vi "Configure Module.vi"(8 "error in (no error)":errorcluster, 10 "IOV ref in":refnum<k21>, 11 "Module Template in":refnum<class "9234.lvclass">) -> (0 "error out":errorcluster, 2 "IOV ref out":refnum<k21>, 3 "Module Template out":refnum<class "9234.lvclass">)   [LabVIEW 2017, in "Modules.lvlib" / "9234.lvclass"]
uses:
  9234.lvclass
  9234.lvclass/9234.ctl
  <resource>/objmgr/cRIO.rc
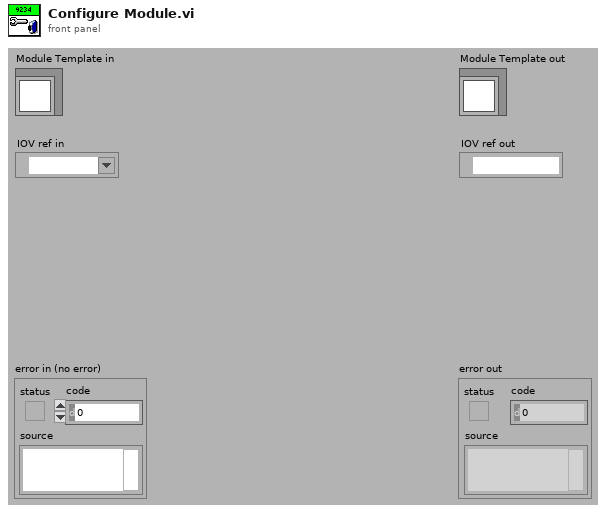
[diagram p1: front panel]
types:
  T1 = typedef "Modules.lvlib/9234.lvclass/Data rate.ctl" = u32
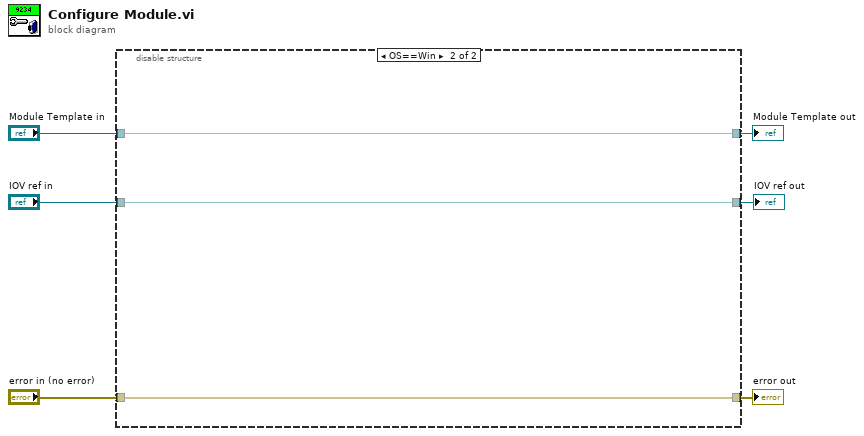
[diagram p0: block diagram]
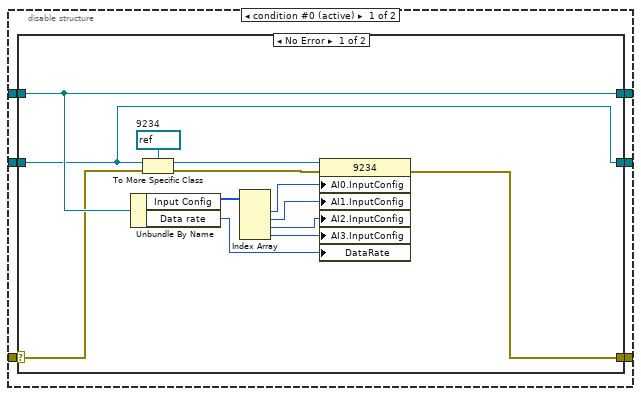
[diagram p2: hidden frame]
diagram:
  n1 = disable-structure shown="OS==Win" {
    disable-tunnel: "error in (no error)" -> [w12 w29]
    disable-tunnel: [w11 w29] -> w5
    disable-tunnel: "Module Template in" -> [w10 w31]
    disable-tunnel: [w9 w31] -> w3
    disable-tunnel: "IOV ref in" -> [w8 w30]
    disable-tunnel: [w7 w30] -> w1
    frame condition #0 (active) {
      n2 = case shown="No Error" w12 {
        selector: w12 -> [w24 w28]
        tunnel: [w20 w28] -> w11
        tunnel: [w25 w27] -> w9
        tunnel: w10 -> [w25 w27]
        tunnel: w8 -> [w19 w26]
        tunnel: [w19 w26] -> w7
        frame No Error {
          w23 = refnum<k21> refnum  # 9234
          n3 = Unbundle By Name(w25) -> ("Input Config"=w18:u32[], "Data rate"=w13:T1)
          n4 = To More Specific Class(target class=w23, reference=w19, error in=w24) -> (specific class reference=w22:refnum<k21>, error out=w21:errorcluster)
          n5 = Index Array(array=w18) -> (element #1=w17:u32, element #2=w16:u32, element #3=w15:u32, element #4=w14:u32)  [unwired: 4 in]
          n6 = property class="9234"(reference=w22, error in=w21, "AI0.InputConfig"=w17, "AI1.InputConfig"=w16, "AI2.InputConfig"=w15, "AI3.InputConfig"=w14, "DataRate"=w13) -> (error out=w20:errorcluster)  [unwired: 1 out]
        }
        frame Error {
        }
      }
    }
    frame condition #1 {
    }
  }
  "error out" <- w5
  "Module Template out" <- w3
  "IOV ref out" <- w1
